vi "Clear Type Map.vi"(8 "error in (no error)":errorcluster, 11 "TwinCAT ADS in":refnum<class "TwinCAT ADS.lvclass">) -> (0 "error out":errorcluster, 2 "[Type Name]":string[](array[string]), 3 "TwinCAT ADS out":refnum<class "TwinCAT ADS.lvclass">)   [LabVIEW 2018, in "TwinCAT ADS.lvclass"]
uses:
  TwinCAT ADS.lvclass
  TwinCAT ADS.lvclass/TwinCAT ADS.ctl
  TwinCAT.Ads
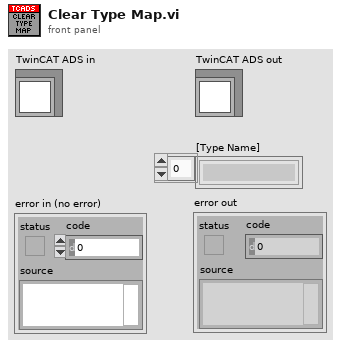
[diagram p1: front panel]
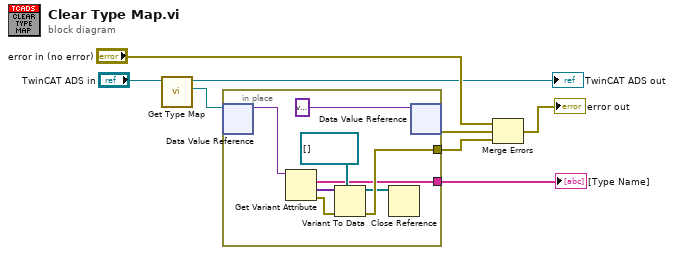
[diagram p0: block diagram]
diagram:
  n1 = call "Get Type Map.vi"("TwinCAT ADS in"="TwinCAT ADS in") -> ("Type Map"=w2:refnum<data-value>, "TwinCAT ADS out"=→"TwinCAT ADS out":refnum<class "TwinCAT ADS.lvclass">)  [unwired: 8 in, 1 out]
  n2 = in-place {
    in-place-border: [w11] -> w8
    in-place-border: [w9] -> w1
    n3 = in-place-dvr #1(w2) -> (w15:variant)  [unwired: 1 out]
    n4 = Get Variant Attribute(Variant=w15) -> (names=w9:string[], values=w13:variant[], error out=w14:errorcluster)  [unwired: 3 in, 1 out]
    n5 = Variant To Data(error in=w14, type=refnum<k24>[] [], Variant=w13) -> (data=w10:refnum<k24>[], error out=w11:errorcluster)
    n6 = Close Reference(reference=w10) -> ()  [unwired: 1 in, 1 out]
    n7 = in-place-dvr #1(variant ("data value")) -> (w7:errorcluster)  [unwired: 1 out]
  }
  "[Type Name]" <- w1
  n8 = Merge Errors("error in (no error)", w7, w8) -> (→"error out":errorcluster)
